vi "note_array.create.vi"(8 "error in":errorcluster, 10 "Events by time":T2(c390), 11 "Px per second":dbl) -> (0 "error out":errorcluster, 3 "Note Array":T1(array[cluster]))   [LabVIEW 2020, in "midi-ui.lvclass"]
uses:
  midi-ui.lvclass
  midi-ui.lvclass/midi-ui.ctl
  midi-file-event.midi/midi-file-event.midi.lvclass
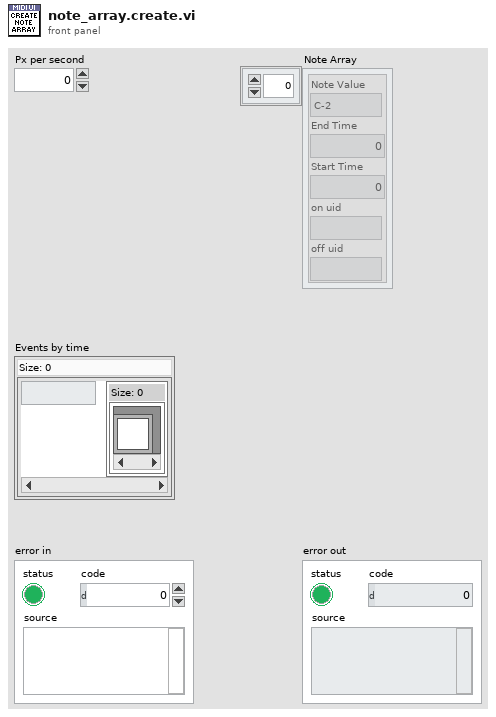
[diagram p1: front panel]
types:
  T1 = cluster{"Note Value":enum8{"C-2", "C#-2", "D-2", "D#-2", "E-2", "F-2", "F#-2", "G-2", "G#-2", "A-2", "A#-2", "B-2", "C-1", "C#-1", "D-1", "D#-1", "E-1", "F-1", "F#-1", "G-1", "G#-1", "A-1", "A#-1", "B-1", "C0", "C#0", "D0", "D#0", "E0", "F0", "F#0", "G0", "G#0", "A0", "A#0", "B0", "C1", "C#1", "D1", "D#1", "E1", "F1", "F#1", "G1", "G#1", "A1", "A#1", "B1", "C2", "C#2", "D2", "D#2", "E2", "F2", "F#2", "G2", "G#2", "A2", "A#2", "B2", "C3", "C#3", "D3", "D#3", "E3", "F3", "F#3", "G3", "G#3", "A3", "A#3", "B3", "C4", "C#4", "D4", "D#4", "E4", "F4", "F#4", "G4", "G#4", "A4", "A#4", "B4", "C5", "C#5", "D5", "D#5", "E5", "F5", "F#5", "G5", "G#5", "A5", "A#5", "B5", "C6", "C#6", "D6", "D#6", "E6", "F6", "F#6", "G6", "G#6", "A6", "A#6", "B6", "C7", "C#7", "D7", "D#7", "E7", "F7", "F#7", "G7", "G#7", "A7", "A#7", "B7", "C8", "C#8", "D8", "D#8", "E8", "F8", "F#8", "G"}, "End Time":u32, "Start Time":u32, "on uid":string, "off uid":string}[]
  T2 = map{dbl, set{refnum<class "midi-file-event.midi.lvclass">}}
  T3 = map{enum8{"C-2", "C#-2", "D-2", "D#-2", "E-2", "F-2", "F#-2", "G-2", "G#-2", "A-2", "A#-2", "B-2", "C-1", "C#-1", "D-1", "D#-1", "E-1", "F-1", "F#-1", "G-1", "G#-1", "A-1", "A#-1", "B-1", "C0", "C#0", "D0", "D#0", "E0", "F0", "F#0", "G0", "G#0", "A0", "A#0", "B0", "C1", "C#1", "D1", "D#1", "E1", "F1", "F#1", "G1", "G#1", "A1", "A#1", "B1", "C2", "C#2", "D2", "D#2", "E2", "F2", "F#2", "G2", "G#2", "A2", "A#2", "B2", "C3", "C#3", "D3", "D#3", "E3", "F3", "F#3", "G3", "G#3", "A3", "A#3", "B3", "C4", "C#4", "D4", "D#4", "E4", "F4", "F#4", "G4", "G#4", "A4", "A#4", "B4", "C5", "C#5", "D5", "D#5", "E5", "F5", "F#5", "G5", "G#5", "A5", "A#5", "B5", "C6", "C#6", "D6", "D#6", "E6", "F6", "F#6", "G6", "G#6", "A6", "A#6", "B6", "C7", "C#7", "D7", "D#7", "E7", "F7", "F#7", "G7", "G#7", "A7", "A#7", "B7", "C8", "C#8", "D8", "D#8", "E8", "F8", "F#8", "G"}, cluster{"Note Value":enum8{"C-2", "C#-2", "D-2", "D#-2", "E-2", "F-2", "F#-2", "G-2", "G#-2", "A-2", "A#-2", "B-2", "C-1", "C#-1", "D-1", "D#-1", "E-1", "F-1", "F#-1", "G-1", "G#-1", "A-1", "A#-1", "B-1", "C0", "C#0", "D0", "D#0", "E0", "F0", "F#0", "G0", "G#0", "A0", "A#0", "B0", "C1", "C#1", "D1", "D#1", "E1", "F1", "F#1", "G1", "G#1", "A1", "A#1", "B1", "C2", "C#2", "D2", "D#2", "E2", "F2", "F#2", "G2", "G#2", "A2", "A#2", "B2", "C3", "C#3", "D3", "D#3", "E3", "F3", "F#3", "G3", "G#3", "A3", "A#3", "B3", "C4", "C#4", "D4", "D#4", "E4", "F4", "F#4", "G4", "G#4", "A4", "A#4", "B4", "C5", "C#5", "D5", "D#5", "E5", "F5", "F#5", "G5", "G#5", "A5", "A#5", "B5", "C6", "C#6", "D6", "D#6", "E6", "F6", "F#6", "G6", "G#6", "A6", "A#6", "B6", "C7", "C#7", "D7", "D#7", "E7", "F7", "F#7", "G7", "G#7", "A7", "A#7", "B7", "C8", "C#8", "D8", "D#8", "E8", "F8", "F#8", "G"}, "End Time":u32, "Start Time":u32, "on uid":string, "off uid":string}}
  T4 = enum8{"C-2", "C#-2", "D-2", "D#-2", "E-2", "F-2", "F#-2", "G-2", "G#-2", "A-2", "A#-2", "B-2", "C-1", "C#-1", "D-1", "D#-1", "E-1", "F-1", "F#-1", "G-1", "G#-1", "A-1", "A#-1", "B-1", "C0", "C#0", "D0", "D#0", "E0", "F0", "F#0", "G0", "G#0", "A0", "A#0", "B0", "C1", "C#1", "D1", "D#1", "E1", "F1", "F#1", "G1", "G#1", "A1", "A#1", "B1", "C2", "C#2", "D2", "D#2", "E2", "F2", "F#2", "G2", "G#2", "A2", "A#2", "B2", "C3", "C#3", "D3", "D#3", "E3", "F3", "F#3", "G3", "G#3", "A3", "A#3", "B3", "C4", "C#4", "D4", "D#4", "E4", "F4", "F#4", "G4", "G#4", "A4", "A#4", "B4", "C5", "C#5", "D5", "D#5", "E5", "F5", "F#5", "G5", "G#5", "A5", "A#5", "B5", "C6", "C#6", "D6", "D#6", "E6", "F6", "F#6", "G6", "G#6", "A6", "A#6", "B6", "C7", "C#7", "D7", "D#7", "E7", "F7", "F#7", "G7", "G#7", "A7", "A#7", "B7", "C8", "C#8", "D8", "D#8", "E8", "F8", "F#8", "G"}
  T5 = cluster{"Note Value":enum8{"C-2", "C#-2", "D-2", "D#-2", "E-2", "F-2", "F#-2", "G-2", "G#-2", "A-2", "A#-2", "B-2", "C-1", "C#-1", "D-1", "D#-1", "E-1", "F-1", "F#-1", "G-1", "G#-1", "A-1", "A#-1", "B-1", "C0", "C#0", "D0", "D#0", "E0", "F0", "F#0", "G0", "G#0", "A0", "A#0", "B0", "C1", "C#1", "D1", "D#1", "E1", "F1", "F#1", "G1", "G#1", "A1", "A#1", "B1", "C2", "C#2", "D2", "D#2", "E2", "F2", "F#2", "G2", "G#2", "A2", "A#2", "B2", "C3", "C#3", "D3", "D#3", "E3", "F3", "F#3", "G3", "G#3", "A3", "A#3", "B3", "C4", "C#4", "D4", "D#4", "E4", "F4", "F#4", "G4", "G#4", "A4", "A#4", "B4", "C5", "C#5", "D5", "D#5", "E5", "F5", "F#5", "G5", "G#5", "A5", "A#5", "B5", "C6", "C#6", "D6", "D#6", "E6", "F6", "F#6", "G6", "G#6", "A6", "A#6", "B6", "C7", "C#7", "D7", "D#7", "E7", "F7", "F#7", "G7", "G#7", "A7", "A#7", "B7", "C8", "C#8", "D8", "D#8", "E8", "F8", "F#8", "G"}, "End Time":u32, "Start Time":u32, "on uid":string, "off uid":string}
  T6 = set{refnum<class "midi-file-event.midi.lvclass">}
  T7 = typedef "midi-file.lvclass/MIDI Messages.ctl" = enum8{"0(0x00)_UnassignedMidiMessage", "1(0x01)_UnassignedMidiMessage", "2(0x02)_UnassignedMidiMessage", "3(0x03)_UnassignedMidiMessage", "4(0x04)_UnassignedMidiMessage", "5(0x05)_UnassignedMidiMessage", "6(0x06)_UnassignedMidiMessage", "7(0x07)_UnassignedMidiMessage", "8(0x08)_NoteOffEvent", "9(0x09)_NoteOnEvent", "10(0x0A)_PolyphonicKeyPressure", "11(0x0B)_ControlChange", "12(0x0C)_ProgramChange", "13(0x0D)_ChannelPressure", "14(0x0E)_PitchBendChange", "15(0x0F)_SystemExclusive(SysEx)", "16(0x10)_UnassignedMidiMessage", "17(0x11)_UnassignedMidiMessage", "18(0x12)_UnassignedMidiMessage", "19(0x13)_UnassignedMidiMessage", "20(0x14)_UnassignedMidiMessage", "21(0x15)_UnassignedMidiMessage", "22(0x16)_UnassignedMidiMessage", "23(0x17)_UnassignedMidiMessage", "24(0x18)_UnassignedMidiMessage", "25(0x19)_UnassignedMidiMessage", "26(0x1A)_UnassignedMidiMessage", "27(0x1B)_UnassignedMidiMessage", "28(0x1C)_UnassignedMidiMessage", "29(0x1D)_UnassignedMidiMessage", "30(0x1E)_UnassignedMidiMessage", "31(0x1F)_UnassignedMidiMessage", "32(0x20)_UnassignedMidiMessage", "33(0x21)_UnassignedMidiMessage", "34(0x22)_UnassignedMidiMessage", "35(0x23)_UnassignedMidiMessage", "36(0x24)_UnassignedMidiMessage", "37(0x25)_UnassignedMidiMessage", "38(0x26)_UnassignedMidiMessage", "39(0x27)_UnassignedMidiMessage", "40(0x28)_UnassignedMidiMessage", "41(0x29)_UnassignedMidiMessage", "42(0x2A)_UnassignedMidiMessage", "43(0x2B)_UnassignedMidiMessage", "44(0x2C)_UnassignedMidiMessage", "45(0x2D)_UnassignedMidiMessage", "46(0x2E)_UnassignedMidiMessage", "47(0x2F)_UnassignedMidiMessage", "48(0x30)_UnassignedMidiMessage", "49(0x31)_UnassignedMidiMessage", "50(0x32)_UnassignedMidiMessage", "51(0x33)_UnassignedMidiMessage", "52(0x34)_UnassignedMidiMessage", "53(0x35)_UnassignedMidiMessage", "54(0x36)_UnassignedMidiMessage", "55(0x37)_UnassignedMidiMessage", "56(0x38)_UnassignedMidiMessage", "57(0x39)_UnassignedMidiMessage", "58(0x3A)_UnassignedMidiMessage", "59(0x3B)_UnassignedMidiMessage", "60(0x3C)_UnassignedMidiMessage", "61(0x3D)_UnassignedMidiMessage", "62(0x3E)_UnassignedMidiMessage", "63(0x3F)_UnassignedMidiMessage", "64(0x40)_UnassignedMidiMessage", "65(0x41)_UnassignedMidiMessage", "66(0x42)_UnassignedMidiMessage", "67(0x43)_UnassignedMidiMessage", "68(0x44)_UnassignedMidiMessage", "69(0x45)_UnassignedMidiMessage", "70(0x46)_UnassignedMidiMessage", "71(0x47)_UnassignedMidiMessage", "72(0x48)_UnassignedMidiMessage", "73(0x49)_UnassignedMidiMessage", "74(0x4A)_UnassignedMidiMessage", "75(0x4B)_UnassignedMidiMessage", "76(0x4C)_UnassignedMidiMessage", "77(0x4D)_UnassignedMidiMessage", "78(0x4E)_UnassignedMidiMessage", "79(0x4F)_UnassignedMidiMessage", "80(0x50)_UnassignedMidiMessage", "81(0x51)_UnassignedMidiMessage", "82(0x52)_UnassignedMidiMessage", "83(0x53)_UnassignedMidiMessage", "84(0x54)_UnassignedMidiMessage", "85(0x55)_UnassignedMidiMessage", "86(0x56)_UnassignedMidiMessage", "87(0x57)_UnassignedMidiMessage", "88(0x58)_UnassignedMidiMessage", "89(0x59)_UnassignedMidiMessage", "90(0x5A)_UnassignedMidiMessage", "91(0x5B)_UnassignedMidiMessage", "92(0x5C)_UnassignedMidiMessage", "93(0x5D)_UnassignedMidiMessage", "94(0x5E)_UnassignedMidiMessage", "95(0x5F)_UnassignedMidiMessage", "96(0x60)_UnassignedMidiMessage", "97(0x61)_UnassignedMidiMessage", "98(0x62)_UnassignedMidiMessage", "99(0x63)_UnassignedMidiMessage", "100(0x64)_UnassignedMidiMessage", "101(0x65)_UnassignedMidiMessage", "102(0x66)_UnassignedMidiMessage", "103(0x67)_UnassignedMidiMessage", "104(0x68)_UnassignedMidiMessage", "105(0x69)_UnassignedMidiMessage", "106(0x6A)_UnassignedMidiMessage", "107(0x6B)_UnassignedMidiMessage", "108(0x6C)_UnassignedMidiMessage", "109(0x6D)_UnassignedMidiMessage", "110(0x6E)_UnassignedMidiMessage", "111(0x6F)_UnassignedMidiMessage", "112(0x70)_UnassignedMidiMessage", "113(0x71)_UnassignedMidiMessage", "114(0x72)_UnassignedMidiMessage", "115(0x73)_UnassignedMidiMessage", "116(0x74)_UnassignedMidiMessage", "117(0x75)_UnassignedMidiMessage", "118(0x76)_UnassignedMidiMessage", "119(0x77)_UnassignedMidiMessage", "120(0x78)_UnassignedMidiMessage", "121(0x79)_UnassignedMidiMessage", "122(0x7A)_UnassignedMidiMessage", "123(0x7B)_UnassignedMidiMessage", "124(0x7C)_UnassignedMidiMessage", "125(0x7D)_UnassignedMidiMessage", "126(0x7E)_UnassignedMidiMessage", "127(0x7F)_UnassignedMidiMessage"}
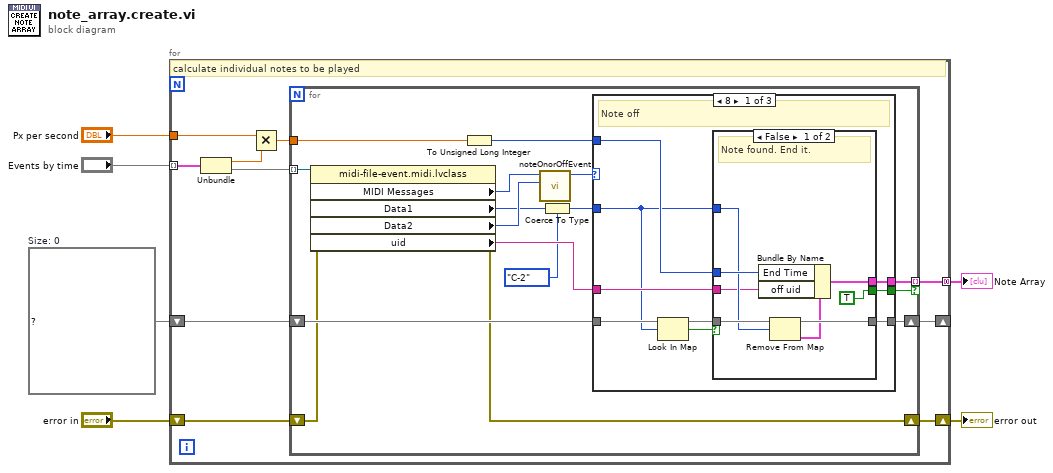
[diagram p0: block diagram]
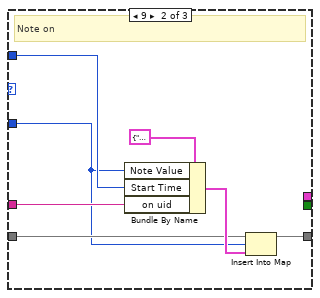
[diagram p3: hidden frame]
diagram:
  w6 = T3 {}  # Size: 0
  n1 = for {
    tunnel: "Events by time" -> [w12] mode=indexing
    shift-right: [w15] -> _
    shift-left: w6 -> [w16]
    tunnel: [w14] -> w3 mode=concatenating
    tunnel: "Px per second" -> [w13]
    shift-right: [w7] -> w1
    shift-left: "error in" -> [w8]
    # "calculate individual notes to be played"
    n2 = Unbundle(w12) -> ("Timestamp"=w11:dbl, w10:T6)
    n3 = Multiply(x=w13, y=w11) -> (x*y=w9:dbl)
    n4 = for {
      tunnel: w9 -> [w30]
      tunnel: [w29] -> w14 mode=indexing if=w22
      tunnel: w10 -> [w23] mode=indexing
      shift-right: [w31] -> w15
      shift-left: w16 -> [w32]
      shift-right: [w17] -> w7
      shift-left: w8 -> [w18]
      n5 = property class="midi-file-event.midi.lvclass"(reference=w23, error in=w18) -> (error out=w17:errorcluster, "MIDI Messages"=w26:T7, "Data1"=w21:u8, "Data2"=w25:u8, "uid"=w24:string)  [unwired: 1 out]
      n6 = To Unsigned Long Integer(number=w30) -> (unsigned 32bit integer=w27:u32)
      n7 = call "noteOnorOffEvent.vi"("Volume"=w25, "MIDI Message"=w26) -> ("Midi Message"=w28:u16)  [unwired: 9 in]
      n8 = Coerce To Type(0:w21, 1:T4."C-2" ("Note Value")) -> (2:w20:T4)
      n9 = case shown="8" w28 {
        tunnel: w32 -> [w36 w52 w57]
        tunnel: [w40 w55 w57] -> w31
        tunnel: w20 -> [w33 w50 _]
        tunnel: w27 -> [w39 w56 _]
        tunnel: [w38 _ _] -> w29
        tunnel: [w37 _ _] -> w22
        tunnel: w24 -> [w34 w53 _]
        frame 8 {
          # "Note off"
          n10 = Look In Map(map=w36, key=w33) -> (key not found?=w35:bool)  [unwired: 1 in, 1 out]
          n11 = case shown="False" w35 {
            tunnel: [w44 w49] -> w40
            tunnel: w36 -> [w45 w49]
            tunnel: w39 -> [w48 _]
            tunnel: [w47 _] -> w38
            tunnel: [TRUE _] -> w37
            tunnel: w33 -> [w43 _]
            tunnel: w34 -> [w41 _]
            frame False {
              # "Note found. End it."
              n12 = Remove From Map(10:w43, 11:w45) -> (1:w42:T5, 3:w44:T3)  [unwired: 1 out]
              n13 = Bundle By Name(cluster=w42, "End Time"=w48, "off uid"=w41) -> (w47:T5)
            }
            frame True {
              # "Not found so ignore"
            }
          }
        }
        frame 9 {
          # "Note on"
          n14 = Bundle By Name(cluster=T5 {"Note Value"=enum."C-2", "End Time"=0, "Start Time"=0, "on uid"="", "off uid"=""}, "Note Value"=w50, "Start Time"=w56, "on uid"=w53) -> (w54:T5)
          n15 = Insert Into Map(map in=w52, key=w50, value=w54) -> (map out=w55:T3)  [unwired: 2 out]
        }
        frame Default {
        }
      }
    }
  }
  "Note Array" <- w3
  "error out" <- w1
